vi "find_ref_test.vi"() -> ()   [LabVIEW 2011]
uses:
  <vilib>/Motion/FlexMotion/CustomControls/CustomControls.llb/AxisOrVectorSpaceControl To Control.flx
panel:
  out "Position (inch)":dbl
  out "Position (steps)":i32
  in  "Search Type":T1(ring)=enum."Reverse Limit"
  in  "Axis or Vector Space":T2 items=["Axis Control"=0, "Axis 1"=1, "Axis 2"=2, "Axis 3"=3, "Axis 4"=4, "Axis 5"=5, "Axis 6"=6, "Axis 7"=7, "Axis 8"=8, "Vector Space Control"=16, "Vector Space 1"=17, "Vector Space 2"=18, "Vector Space 3"=19, "Vector Space 4"=20]
  in  "Board ID":T3=1 min=1 max=32 step=1
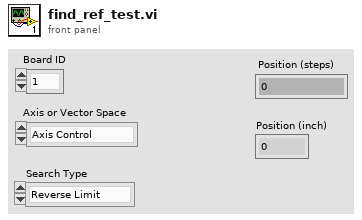
[diagram p1: front panel]
types:
  T1 = enum16{"Home", "Index", "Center", "Forward Limit", "Reverse Limit", "Run Sequence"}
  T2 = typedef "AxisOrVectorSpaceControl To Control.flx" = u16
  T3 = typedef "Board Id" = u8
  T4 = typedef "Bd Id Out" = u8
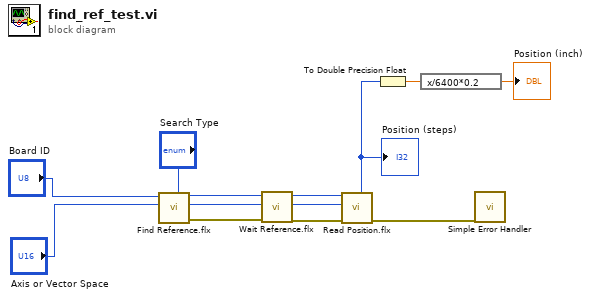
[diagram p0: block diagram]
diagram:
  n1 = call <vilib>:"Find Reference.flx"("Search Type"="Search Type", "Axis or Vector Space"="Axis or Vector Space", "Board ID"="Board ID") -> ("error out"=w10:errorcluster, "Axis or Vector Space Output"=w9:T2, "Bd ID Out"=w8:T4)  [unwired: 6 in]
  n2 = call <vilib>:"Wait Reference.flx"("error in (no error)"=w10, "Axis or Vector Space"=w9, "Board ID"=w8) -> ("error out"=w7:errorcluster, "Axis or Vector Space Output"=w6:T2, "Bd ID Out"=w5:T4)  [unwired: 5 in, 1 out]
  n3 = call <vilib>:"Read Position.flx"("error in (no error)"=w7, "Axis"=w6, "Board ID"=w5) -> ("error out"=w4:errorcluster, "Position"=w1:i32)  [unwired: 3 in, 2 out]
  "Position (steps)" <- w1
  n4 = To Double Precision Float(number=w1) -> (double precision float=w2:dbl)
  n5 = expression code="x/6400*0.2"(w2) -> (→"Position (inch)":dbl)
  n6 = call <vilib>:"Simple Error Handler.vi"("error in (no error)"=w4) -> ()  [unwired: 4 in, 5 out]
